vi "enableZeroCheck.vi"(8 "error in (no error)":errorcluster, 10 "Enable Zero Check (T: Enable)":bool, 11 "Electrometer in":refnum<class "Electrometer.lvclass">) -> (0 "error out":errorcluster, 3 "Electrometer out":refnum<class "Electrometer.lvclass">)   [LabVIEW 2016, in "Electrometer.lvclass"]
uses:
  Electrometer.lvclass
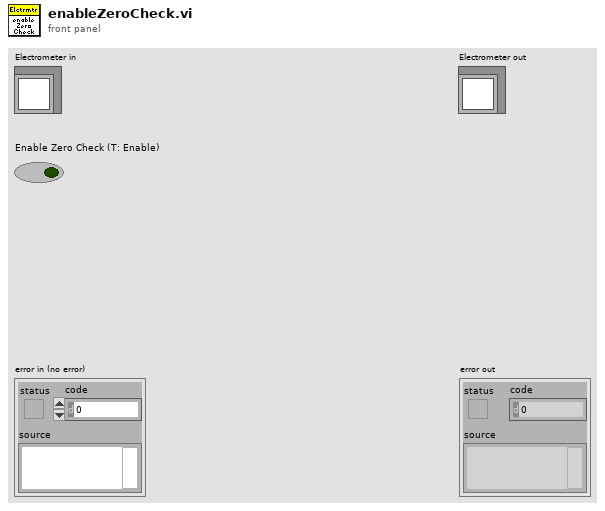
[diagram p1: front panel]
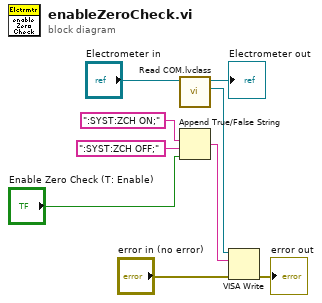
[diagram p0: block diagram]
diagram:
  n1 = call "Read COM.lvclass.vi"("Electrometer in"="Electrometer in") -> ("VISA"=w5:refnum<visa-resource-name>, "Electrometer out"=→"Electrometer out":refnum<class "Electrometer.lvclass">)  [unwired: 8 in, 1 out]
  n2 = Append True/False String(1:"Enable Zero Check (T: Enable)", 2:":SYST:ZCH OFF;", 3:":SYST:ZCH ON;") -> (0:w6:string)  [unwired: 1 in]
  n3 = VISA Write(VISA resource name=w5, write buffer=w6, error in (no error)="error in (no error)") -> (error out=→"error out":errorcluster)  [unwired: 2 out]
